vi "SWERVE_TRAJECTORY_GLOBALS.vi"() -> ()   [LabVIEW 2019]
panel:
  out "Traj Heading Dmd":dbl format="%17.2f"
  out "Traj Y Corr":dbl format="%17.2f"
  out "Traj X Corr":dbl format="%17.2f"
  out "Traj Closed Loop":bool
  out "Traj Curvature Sample":dbl format="%17.2f"
  out "Traj Velocity Sample":dbl format="%17.2f"
  out "Traj Heading Sample":dbl format="%17.2f"
  out "Traj Y Sample":dbl format="%17.2f"
  out "Traj X Sample":dbl format="%17.2f"
  out "Traj_IsGood":bool
  out "Traj_Total_Time":dbl format="%17.2f"
  out "Traj_Total_States":dbl format="%17.2f"
  out "Traj Heading Err":dbl format="%17.2f"
  out "Traj Y Err":dbl format="%17.2f"
  out "Traj X Err":dbl format="%17.2f"
  out "Traj_OnTarget":bool
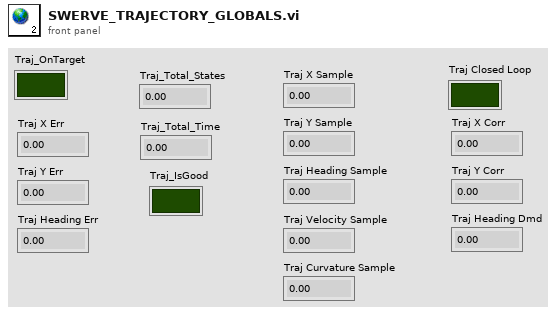
[diagram p1: front panel]
diagram:
